vi "Tabor 5064 - Set Channel Output State (SubVI).vi"(6 "write_delay (ms)":u32=100, 7 "GPIB Address":string="4", 8 "error_in":errorcluster, 11 "ch_enable":bool[](array[boolean])=[FALSE, FALSE, FALSE, FALSE]) -> (0 "error_out":errorcluster)   [LabVIEW 2022 SP3]
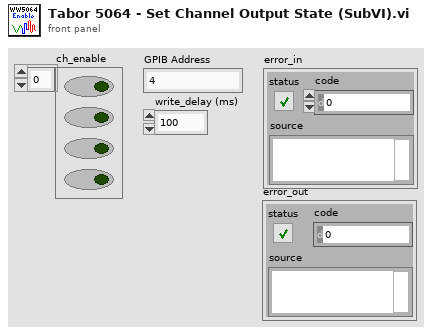
[diagram p1: front panel]
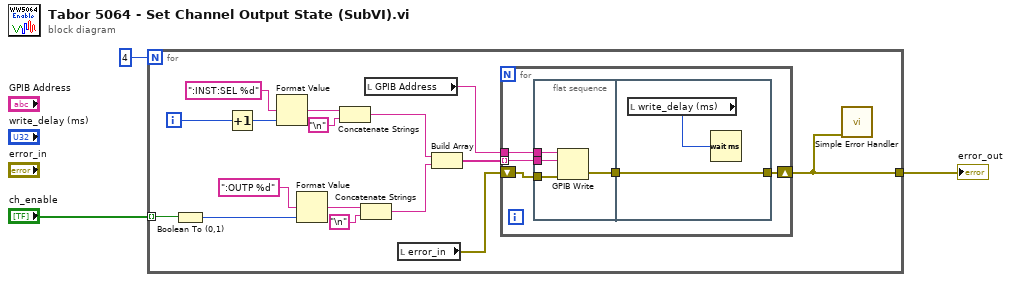
[diagram p0: block diagram]
diagram:
  n1 = for {
    N: 4 -> [_]
    tunnel: "ch_enable" -> [w7] mode=indexing
    tunnel: [w5] -> w1
    i -> [w10]
    n2 = Boolean To (0,1)(Boolean=w7) -> (0, 1=w8:i16)
    n3 = Increment(x=w10) -> (x+1=w18:i32)
    n4 = Format Value(format string=":INST:SEL %d", value (0)=w18) -> (output string=w19:string)  [unwired: 1 in]
    n5 = Format Value(format string=":OUTP %d", value (0)=w8) -> (output string=w13:string)  [unwired: 1 in]
    n6 = Concatenate Strings(w19, "\n") -> (w12:string)
    n7 = Concatenate Strings(w13, "\n") -> (w11:string)
    n8 = local read "GPIB Address"() -> (w6:string)
    n9 = local read "error_in"() -> (w4:errorcluster)
    n10 = Build Array(w12, w11) -> (w9:string[])
    n11 = for {
      tunnel: w6 -> [w24]
      tunnel: w9 -> [w23] mode=indexing
      shift-right: [w22] -> w5
      shift-left: w4 -> [w21]
      n12 = flat-sequence {
        tunnel: w24 -> [w28]
        tunnel: w23 -> [w27]
        tunnel: w21 -> [w25]
        tunnel: [w26] -> w20
        tunnel: [w30] -> w22
        tunnel: w20 -> [w30]
        frame #0 {
          n13 = GPIB Write(0:w28, 1:w27, 3:w25) -> (6:w26:errorcluster)  [unwired: 2 in, 1 out]
        }
        frame #1 {
          n14 = local read "write_delay (ms)"() -> (w29:u32)
          n15 = Wait (ms)(milliseconds to wait=w29) -> ()  [unwired: 1 out]
        }
      }
    }
    n16 = call <vilib>:"Simple Error Handler.vi"("error in (no error)"=w5) -> ()  [unwired: 4 in, 5 out]
  }
  "error_out" <- w1
